vi "png read demo.vi"() -> ()   [LabVIEW 2013]
doc: "This is a demo to png read\nA none standard png file can show by add a black mask.\nThe molly.png show a story about 上海地铁女侠"
panel:
  out "without alpha":picture
  out "molly":picture
  out "with alpha":picture
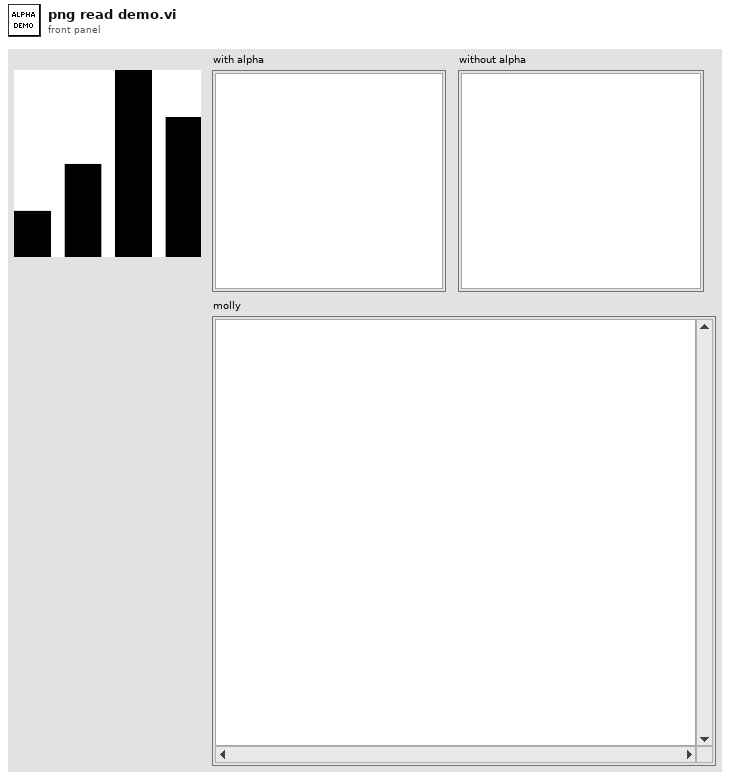
[diagram p1: front panel]
types:
  T1 = typedef "imagedata.ctl" = cluster{"image type":i32, "image depth":i32, "image":u8[], "mask":u8[], "colors":u32[], "Rectangle":cluster{"left":i16, "top":i16, "right":i16, "bottom":i16}}
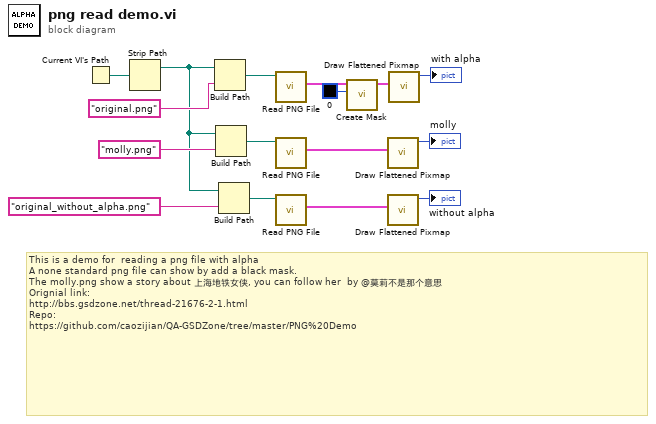
[diagram p0: block diagram]
diagram:
  # "This is a demo for  reading a png file with alpha \nA none standard png file can show by add a black mask.\nThe molly.png show a story about 上海地铁女侠, you can follow her  by @莫莉不是那个意思\nOrignial link:\nhttp://bbs.gsdzone.net/thread-21676-2-1.html\nRepo:\nhttps://github.com/caozijian/QA-GSDZone/tree/master/PNG%20Demo"
  n1 = Current VI's Path() -> (path=w16:path)
  n2 = Strip Path(path=w16) -> (stripped path=w8:path)  [unwired: 1 out]
  n3 = Build Path(base path=w8, name or relative path="original.png") -> (appended path=w13:path)
  n4 = Build Path(base path=w8, name or relative path="molly.png") -> (appended path=w6:path)
  n5 = Build Path(base path=w8, name or relative path="original_without_alpha.png") -> (appended path=w5:path)
  n6 = call <vilib>:"Read PNG File.vi"("path to PNG file"=w13) -> ("image data"=w4:T1)  [unwired: 8 in, 2 out]
  n7 = call <vilib>:"Read PNG File.vi"("path to PNG file"=w6) -> ("image data"=w12:T1)  [unwired: 8 in, 2 out]
  n8 = call <vilib>:"Read PNG File.vi"("path to PNG file"=w5) -> ("image data"=w2:T1)  [unwired: 8 in, 2 out]
  n9 = call <vilib>:"Create Mask.vi"("Mask Color (Black)"=u32 0, "image data"=w4) -> ("image data"=w3:T1)  [unwired: 9 in]
  n10 = call <vilib>:"Draw Flattened Pixmap.vi"("image data"=w12) -> ("new picture"=→"molly":picture)  [unwired: 8 in]
  n11 = call <vilib>:"Draw Flattened Pixmap.vi"("image data"=w2) -> ("new picture"=→"without alpha":picture)  [unwired: 8 in]
  n12 = call <vilib>:"Draw Flattened Pixmap.vi"("image data"=w3) -> ("new picture"=→"with alpha":picture)  [unwired: 8 in]
